vi "Enum Client.vi"() -> ()   [LabVIEW 2020]
uses:
  source/Client/Subscription/Subscription.lvclass
  source/PV Data/NT Base/NT Base.lvclass
  source/Client/Client/Client.lvclass
  source/Client/Client/Put - NT Enum (Index).vi
  source/Client/Subscription/Next Value - NT Enum.vi
  source/PV Data/NT Enum/NT Enum.lvclass
panel:
  in  "Value":u16(ring) items=["A", "B", "C"]
  in  "stop":bool
  in  "PV name":string="DEV:ENUM1"
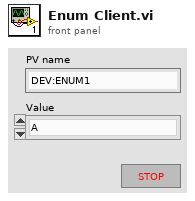
[diagram p1: front panel]
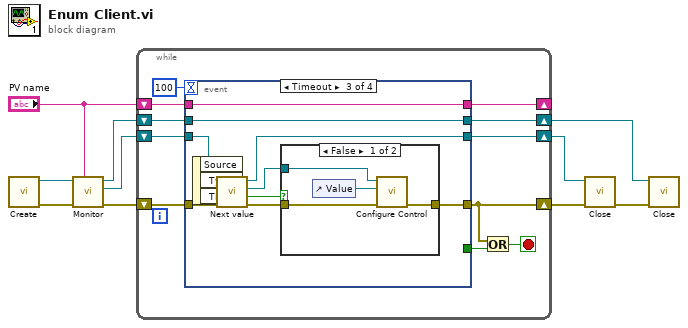
[diagram p0: block diagram]
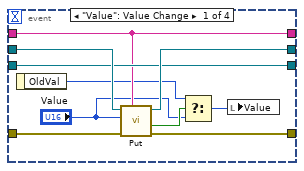
[diagram p2: hidden frame]
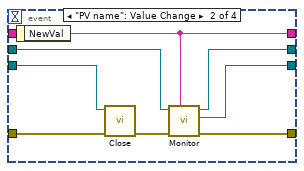
[diagram p3: hidden frame]
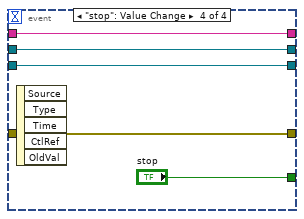
[diagram p5: hidden frame]
diagram:
  n1 = call "Create.vi"() -> ("error out"=w9:errorcluster, "Client out"=w8:refnum<class "Client.lvclass">)  [unwired: 10 in]
  n2 = call "Monitor.vi"("PV name"="PV name", "error in"=w9, "Client in"=w8) -> ("error out"=w5:errorcluster, "subscription"=w4:refnum<class "Subscription.lvclass">, "Client out"=w6:refnum<class "Client.lvclass">)  [unwired: 6 in]
  n3 = while {
    shift-right: [w12] -> w3
    shift-left: w5 -> [w21]
    shift-right: [w20] -> w10
    shift-left: w6 -> [w19]
    shift-right: [w16] -> w2
    shift-left: w4 -> [w17]
    shift-right: [w11] -> _
    shift-left: "PV name" -> [w18]
    stop <- w13 stop-if-true
    n4 = event shown="[2] Timeout" {
      selector: _ -> [_ _ _ _]
      dyn-events: _ -> [_ _ _ _]
      timeout: 100 -> [_ _ _ _]
      tunnel: [_ _ _ "stop"] -> w14
      tunnel: w21 -> [w31 w39 w48 w56]
      tunnel: [w30 w33 w44 w56] -> w12
      tunnel: [w29 w36 w42 w57] -> w20
      tunnel: w19 -> [w28 w35 w42 w57]
      tunnel: w18 -> [w26 _ w40 w54]
      tunnel: w17 -> [w27 w38 w47 w55]
      tunnel: [w27 w37 w43 w55] -> w16
      tunnel: [w26 w32 w40 w54] -> w11
      event "Value": Value Change {
        n5 = event-data() -> ("OldVal"=w23:u16)  [unwired: 1 in]
        n6 = call-poly "Put.vi"("PV name"=w26, "error in (no error)"=w31, "index"="Value", "Client in"=w28) -> ("error out"=w30:errorcluster, "timed out?"=w25:bool, "Client out"=w29:refnum<class "Client.lvclass">)  [unwired: 5 in]
        n7 = Select(t=w23, s=w25, f="Value") -> (s? t:f=w24:u16)
        n8 = local write "Value"(w24) -> ()
      }
      event "PV name": Value Change {
        n9 = event-data() -> ("NewVal"=w32:string)  [unwired: 1 in]
        n10 = call-dynamic "Close.vi"("error in (no error)"=w39, "Subscription in"=w38) -> ("error out"=w34:errorcluster)  [unwired: 9 in]
        n11 = call "Monitor.vi"("PV name"=w32, "error in"=w34, "Client in"=w35) -> ("error out"=w33:errorcluster, "subscription"=w37:refnum<class "Subscription.lvclass">, "Client out"=w36:refnum<class "Client.lvclass">)  [unwired: 6 in]
      }
      event Timeout {
        n12 = event-data() -> ()  [unwired: 1 in, 3 out]
        n13 = call-poly "Next value.vi"("error in (no error)"=w48, "Subscription in"=w47) -> ("error out"=w45:errorcluster, "timed out?"=w41:bool, "value"=w46:refnum<class "NT Enum.lvclass">, "Subscription out"=w43:refnum<class "Subscription.lvclass">)  [unwired: 5 in, 1 out]
        n14 = case shown="False" w41 {
          tunnel: w46 -> [w52 _]
          tunnel: w45 -> [w51 w53]
          tunnel: [w50 w53] -> w44
          frame False {
            n15 = control-ref of="Value"() -> (w49:refnum<vi>)
            n16 = call-dynamic "Configure Control.vi"("error in (no error)"=w51, "control"=w49, "NT Enum in"=w52) -> ("error out"=w50:errorcluster)  [unwired: 6 in, 2 out]
          }
          frame True {
          }
        }
      }
      event "stop": Value Change {
        n17 = event-data() -> ()  [unwired: 1 in, 5 out]
      }
    }
    n18 = Or(x=w12, y=w14) -> (x .or. y?=w13:bool)
  }
  n19 = call-dynamic "Close.vi"("error in (no error)"=w3, "Subscription in"=w2) -> ("error out"=w1:errorcluster)  [unwired: 9 in]
  n20 = call "Close.vi"("error in (no error)"=w1, "Client in"=w10) -> ()  [unwired: 9 in, 1 out]
